vi "Heart beat.vi"() -> ()   [LabVIEW 2022 SP3]
uses:
  <vilib>/DAQmx/read.llb/DAQmx Read (Analog DBL 1Chan 1Samp).vi
  <vilib>/DAQmx/create/channels.llb/DAQmx Create Channel (AI-Voltage-Basic).vi
  <vilib>/DAQmx/miscellaneous.llb/DAQmx Fill In Error Info.vi
panel:
  out "BPM":dbl
  out "Count":dbl
  out "time":dbl
  in  "Reset":bool
  in  "physical channels":tag
  out "Waveform Chart":dbl(graph)
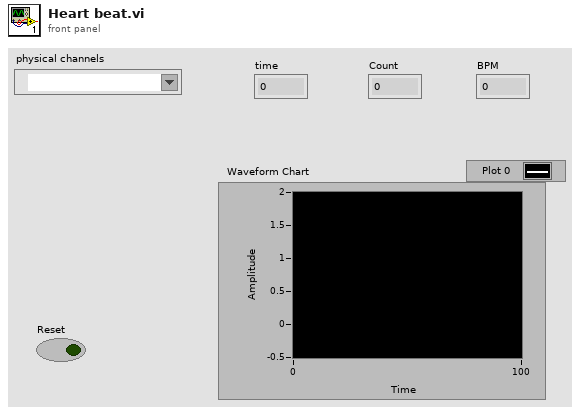
[diagram p1: front panel]
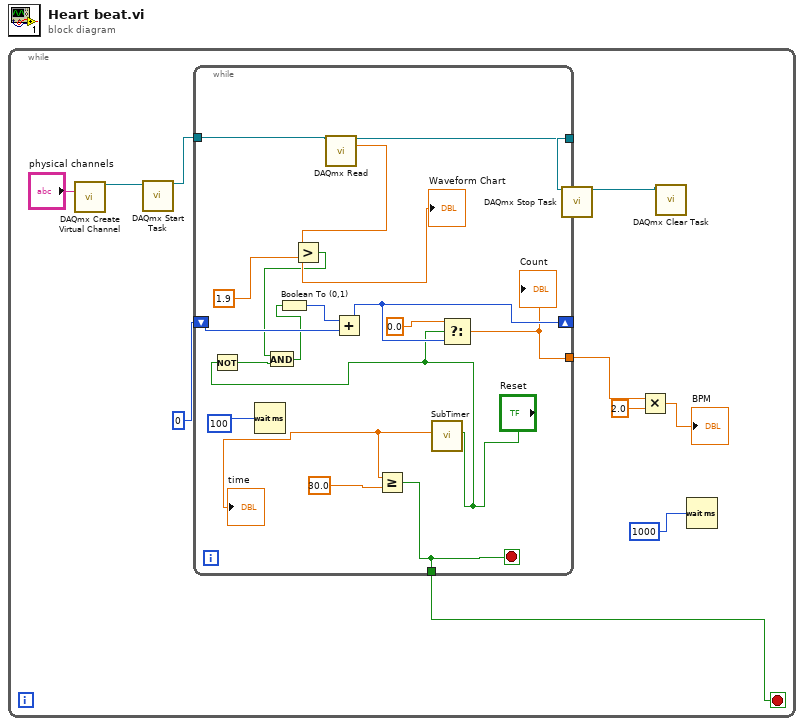
[diagram p0: block diagram]
diagram:
  n1 = while {
    stop <- w1 stop-if-true
    n2 = call-poly <vilib>:"DAQmx Create Virtual Channel.vi"("physical channels"="physical channels") -> ("task out"=w11:refnum<k21>)  [unwired: 13 in, 1 out]
    n3 = call <vilib>:"DAQmx Start Task.vi"("task/channels in"=w11) -> ("task out"=w10:refnum<k21>)  [unwired: 13 in, 1 out]
    n4 = while {
      tunnel: w10 -> [w28]
      tunnel: [w27] -> w9
      shift-right: [w19] -> _
      shift-left: i16 0 -> [w21]
      tunnel: [w13] -> w5
      tunnel: [w12] -> w1
      stop <- w12 stop-if-true
      n5 = Not(x="Reset") -> (.not. x?=w15:bool)
      n6 = Wait (ms)(milliseconds to wait=u32 100) -> ()  [unwired: 1 out]
      n7 = call-poly <vilib>:"DAQmx Read.vi"("task/channels in"=w28) -> ("task out"=w27:refnum<k21>, "data"=w26:dbl)  [unwired: 12 in, 1 out]
      "Waveform Chart" <- w26
      n8 = Greater?(x=w26, y=1.9) -> (0:w17:bool)
      n9 = And(x=w17, y=w15) -> (x .and. y?=w18:bool)
      n10 = Boolean To (0,1)(Boolean=w18) -> (0, 1=w22:i16)
      n11 = Add(x=w22, y=w21) -> (x+y=w19:i16)
      n12 = call "SubTimer.vi"("s"="Reset") -> ("t"=w24:dbl)  [unwired: 10 in]
      "time" <- w24
      n13 = Greater Or Equal?(x=w24, y=30.0) -> (x >= y?=w12:bool)
      n14 = Select(t=0.0, s="Reset", f=w19) -> (s? t:f=w13:dbl)
      "Count" <- w13
    }
    n15 = call <vilib>:"DAQmx Stop Task.vi"("task/channels in"=w9) -> ("task out"=w8:refnum<k21>)  [unwired: 13 in, 1 out]
    n16 = Multiply(x=w5, y=2.0) -> (x*y=→"BPM":dbl)
    n17 = call <vilib>:"DAQmx Clear Task.vi"("task in"=w8) -> ()  [unwired: 14 in, 1 out]
    n18 = Wait (ms)(milliseconds to wait=u32 1000) -> ()  [unwired: 1 out]
  }
